vi "Depth Control.vi"(8 "Current Run No.":u8, 9 "Depth Offset":dbl format="%#_g%%", 10 "Depth Array":dbl[](array[numeric]), 11 "z Cluster":cluster{"zi":dbl, "zp_true":dbl}) -> (1 "zp_work":dbl, 3 "Schedule Depth & Speed":cluster{"Next Depth":dbl, "Current Depth":dbl} {"Current Depth" format="%#_g%%"; "Next Depth" format="%#_g%%"})   [LabVIEW 2016]
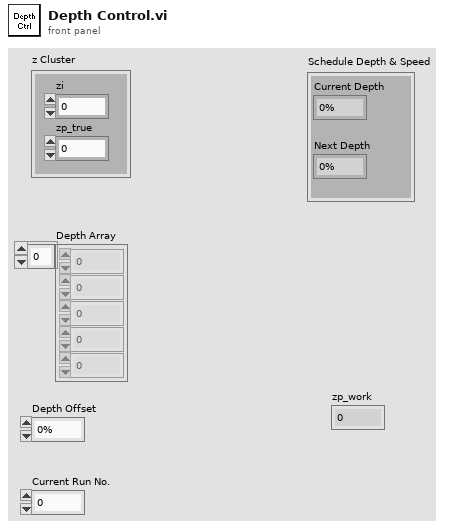
[diagram p1: front panel]
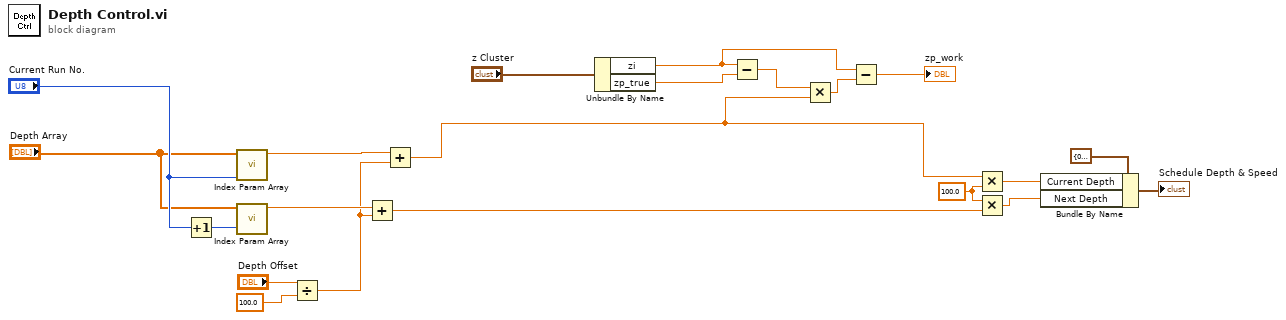
[diagram p0: block diagram]
diagram:
  w8 = 100.0 ("y")
  n1 = Increment(x="Current Run No.") -> (x+1=w20:u8)
  n2 = call "Index Param Array.vi"("Index"="Current Run No.", "Array Input"="Depth Array") -> ("Index Output"=w17:dbl)  [unwired: 9 in]
  n3 = call "Index Param Array.vi"("Index"=w20, "Array Input"="Depth Array") -> ("Index Output"=w19:dbl)  [unwired: 9 in]
  n4 = Divide(x="Depth Offset", y=100.0) -> (x/y=w11:dbl)
  n5 = Add(x=w19, y=w11) -> (x+y=w6:dbl)
  n6 = Add(x=w17, y=w11) -> (x+y=w1:dbl)
  n7 = Unbundle By Name("z Cluster") -> ("zi"=w2:dbl, "zp_true"=w5:dbl)
  n8 = Subtract(x=w2, y=w5) -> (x-y=w4:dbl)
  n9 = Multiply(x=w4, y=w1) -> (x*y=w3:dbl)
  n10 = Subtract(x=w2, y=w3) -> (x-y=→"zp_work":dbl)
  n11 = Multiply(x=w1, y=w8) -> (x*y=w9:dbl)
  n12 = Multiply(x=w8, y=w6) -> (x*y=w7:dbl)
  n13 = Bundle By Name(cluster=cluster{"Next Depth":dbl, "Current Depth":dbl} {"Next Depth"=0.7, "Current Depth"=0.7} ("Schedule Depth & Speed"), "Current Depth"=w9, "Next Depth"=w7) -> (→"Schedule Depth & Speed":cluster{"Next Depth":dbl, "Current Depth":dbl})
